vi "Get Aircraft Attitude.vi"(8 "Error In":errorcluster, 11 "Aircraft ID":u8) -> (0 "Error Out":errorcluster, 3 "Aircraft Att Data Out":T1)   [LabVIEW 2014]
uses:
  Controls/Aircraft Attitude Data.ctl
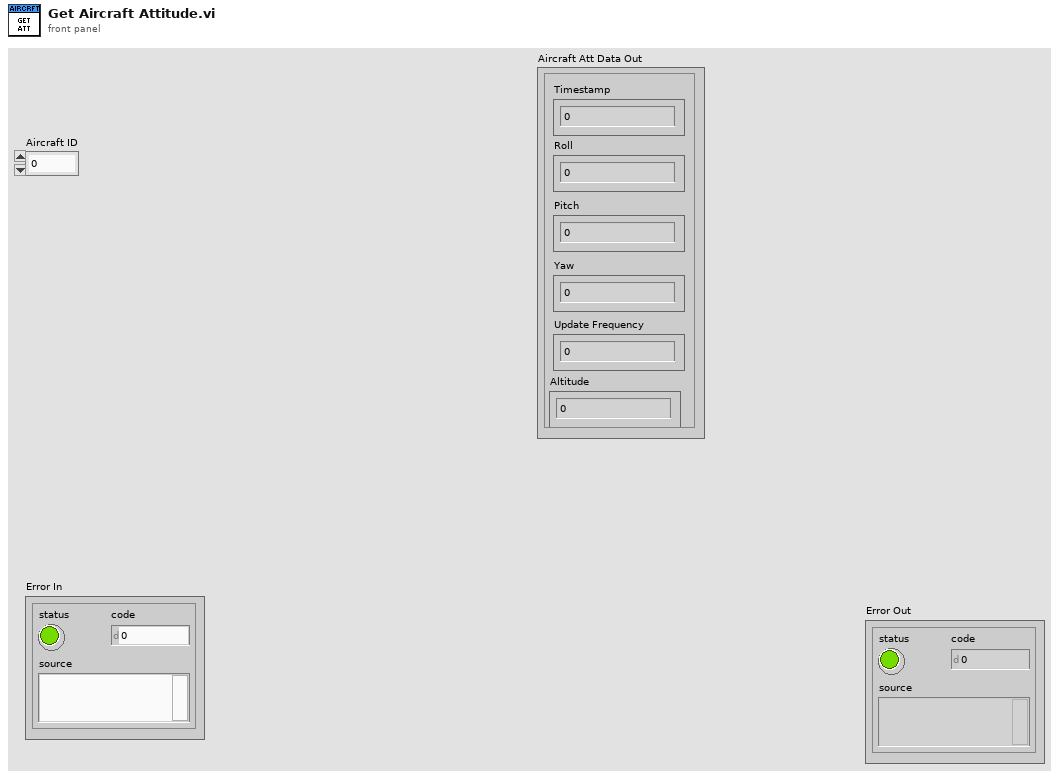
[diagram p1: front panel]
types:
  T1 = typedef "Aircraft Attitude Data.ctl" = cluster{"Roll":sgl, "Pitch":sgl, "Yaw":sgl, "Timestamp":u32, "Update Frequency":dbl, "Altitude":sgl}
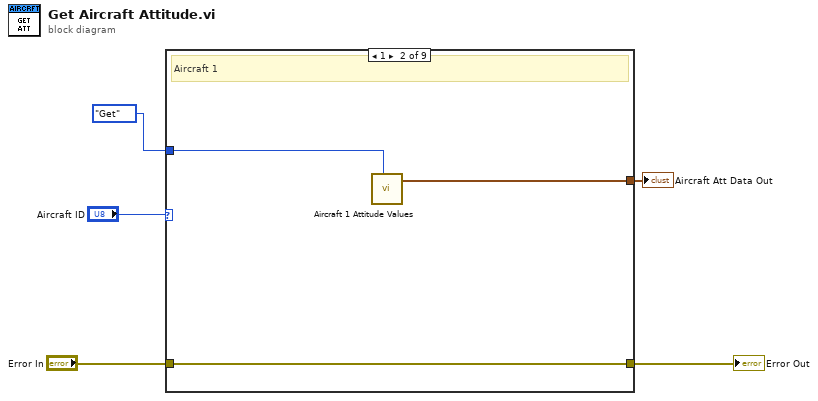
[diagram p0: block diagram]
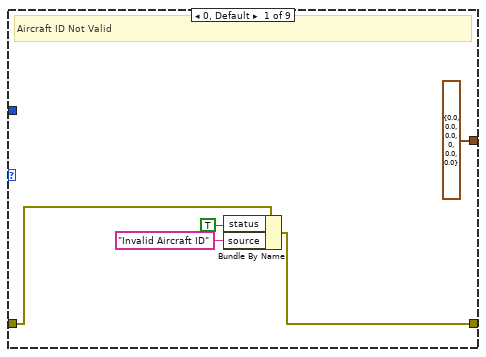
[diagram p2: hidden frame]
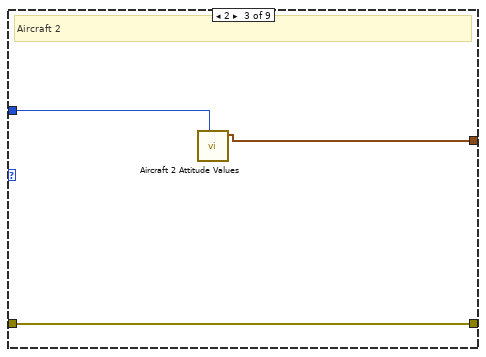
[diagram p3: hidden frame]
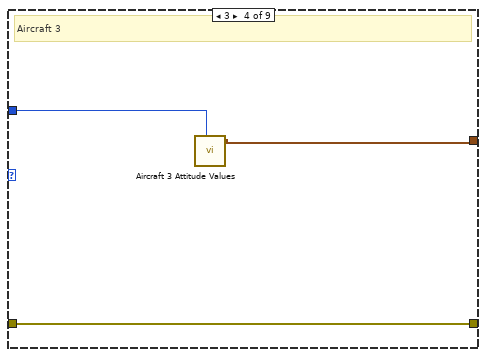
[diagram p4: hidden frame]
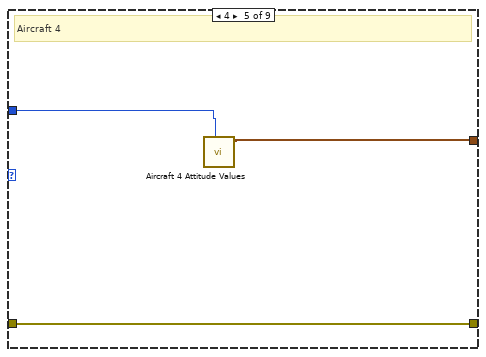
[diagram p5: hidden frame]
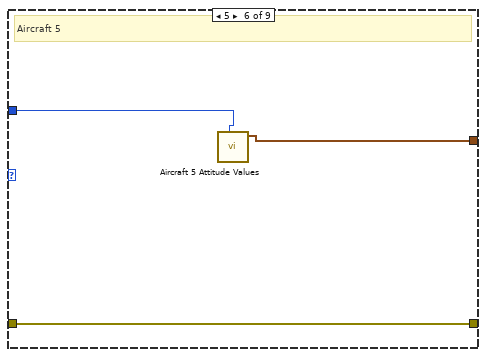
[diagram p6: hidden frame]
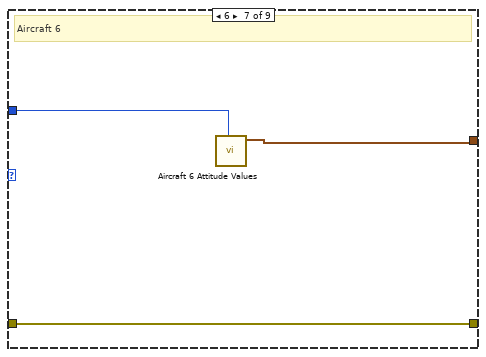
[diagram p7: hidden frame]
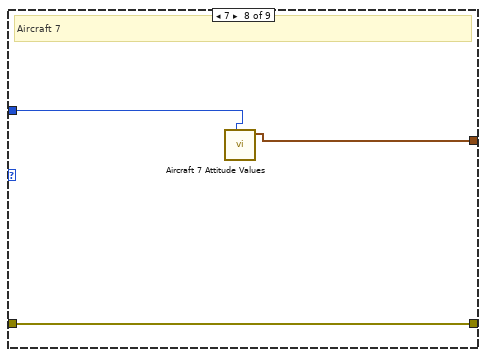
[diagram p8: hidden frame]
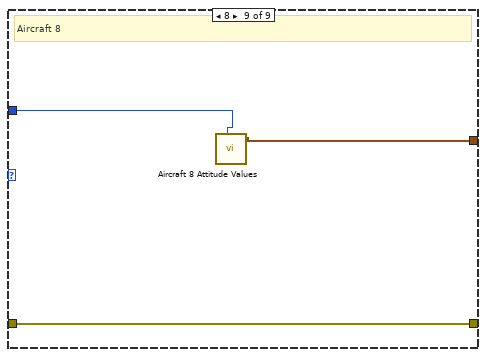
[diagram p9: hidden frame]
diagram:
  n1 = case shown="1" "Aircraft ID" {
    tunnel: [T1 {"Roll"=0.0, "Pitch"=0.0, "Yaw"=0.0, "Timestamp"=0, "Update Frequency"=0.0, "Altitude"=0.0} ("Aircraft Att Data Out") w11 w15 w18 w21 w24 w27 w30 w33] -> w1
    tunnel: [w9 w13 w16 w19 w22 w25 w28 w31 w34] -> w4
    tunnel: "Error In" -> [w10 w13 w16 w19 w22 w25 w28 w31 w34]
    tunnel: enum16{"Get", "Set"}."Get" ("Method") -> [_ w12 w14 w17 w20 w23 w26 w29 w32]
    frame 0, Default {
      # "Aircraft ID Not Valid"
      n2 = Bundle By Name(cluster=w10, "status"=TRUE, "source"="Invalid Aircraft ID") -> (w9:errorcluster)
    }
    frame 1 {
      # "Aircraft 1"
      n3 = call "Aircraft 1 Attitude Values .vi"("Method"=w12) -> ("Aircraft Att Data Out"=w11:T1)  [unwired: 10 in]
    }
    frame 2 {
      # "Aircraft 2"
      n4 = call "Aircraft 2 Attitude Values .vi"("Method"=w14) -> ("Aircraft Att Data Out"=w15:T1)  [unwired: 10 in]
    }
    frame 3 {
      # "Aircraft 3"
      n5 = call "Aircraft 3 Attitude Values .vi"("Method"=w17) -> ("Aircraft Att Data Out"=w18:T1)  [unwired: 10 in]
    }
    frame 4 {
      # "Aircraft 4"
      n6 = call "Aircraft 4 Attitude Values .vi"("Method"=w20) -> ("Aircraft Att Data Out"=w21:T1)  [unwired: 10 in]
    }
    frame 5 {
      # "Aircraft 5"
      n7 = call "Aircraft 5 Attitude Values .vi"("Method"=w23) -> ("Aircraft Att Data Out"=w24:T1)  [unwired: 10 in]
    }
    frame 6 {
      # "Aircraft 6"
      n8 = call "Aircraft 6 Attitude Values .vi"("Method"=w26) -> ("Aircraft Att Data Out"=w27:T1)  [unwired: 10 in]
    }
    frame 7 {
      # "Aircraft 7"
      n9 = call "Aircraft 7 Attitude Values .vi"("Method"=w29) -> ("Aircraft Att Data Out"=w30:T1)  [unwired: 10 in]
    }
    frame 8 {
      # "Aircraft 8"
      n10 = call "Aircraft 8 Attitude Values .vi"("Method"=w32) -> ("Aircraft Att Data Out"=w33:T1)  [unwired: 10 in]
    }
  }
  "Error Out" <- w4
  "Aircraft Att Data Out" <- w1
